vi "light sensor.vi"() -> ()   [LabVIEW 2019]
uses:
  <vilib>/MakerHub/LINX/Public/Utilities/Open Serial.vi
  <vilib>/MakerHub/LINX/LMH-LINX.lvlib
panel:
  out "dt":u32
  out "Lux value":dbl(graph)
  out "current 16bit sensor value":u16
  out "I2C Channel (0)":u8=4
  out "Device Name":string
  in  "stop":bool
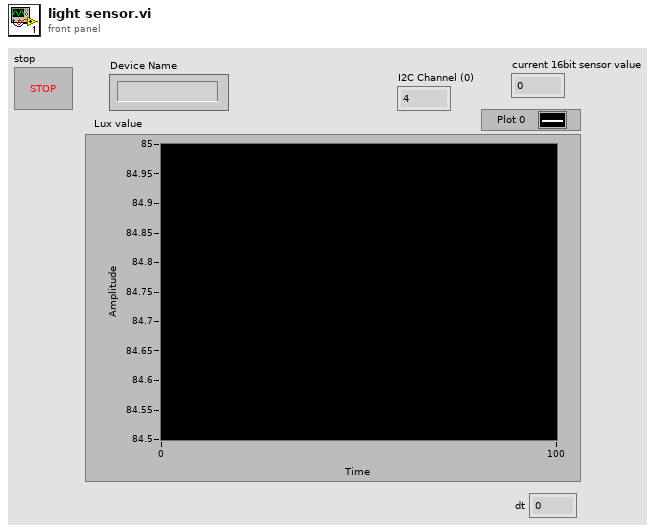
[diagram p1: front panel]
types:
  T1 = typedef "LMH-LINX.lvlib/LINX Ref.ctl" = cluster{"IO":T2, "Interface":T3, "LINX Device Config":T4}
  T2 = typedef "LMH-LINX.lvlib/Platform.ctl" = enum16{"Remote", "Local"}
  T3 = typedef "LMH-LINX.lvlib/Interface.ctl" = enum16{"Serial", "TCP"}
  T4 = typedef "LMH-LINX.lvlib/Device.lvlib/LINX Device Config.ctl" = cluster{"Interface":T3, "COM Port":refnum<visa-resource-name>, "TCP Configuration":T5, "Device Family":u8, "Device ID":u8, "Device Name":string, "TCP Ref":refnum<k5>, "Channels":T6}
  T5 = typedef "LMH-LINX.lvlib/Device.lvlib/TCP Config.ctl" = cluster{"IP Address":string, "Port":u16}
  T6 = typedef "LMH-LINX.lvlib/Channels.ctl" = cluster{"DI":u8[], "DO":u8[], "AI":u8[], "AO":u8[], "PWM":u8[], "QE":u8[], "UART":u8[], "I2C 2":u8[], "SPI":u8[], "CAN":u8[], "Servo":u8[], "AI Ref (V)":dbl, "AI Resolution (Bits)":u8, "AO Ref (V)":dbl, "AO Resolution (Bits)":u8}
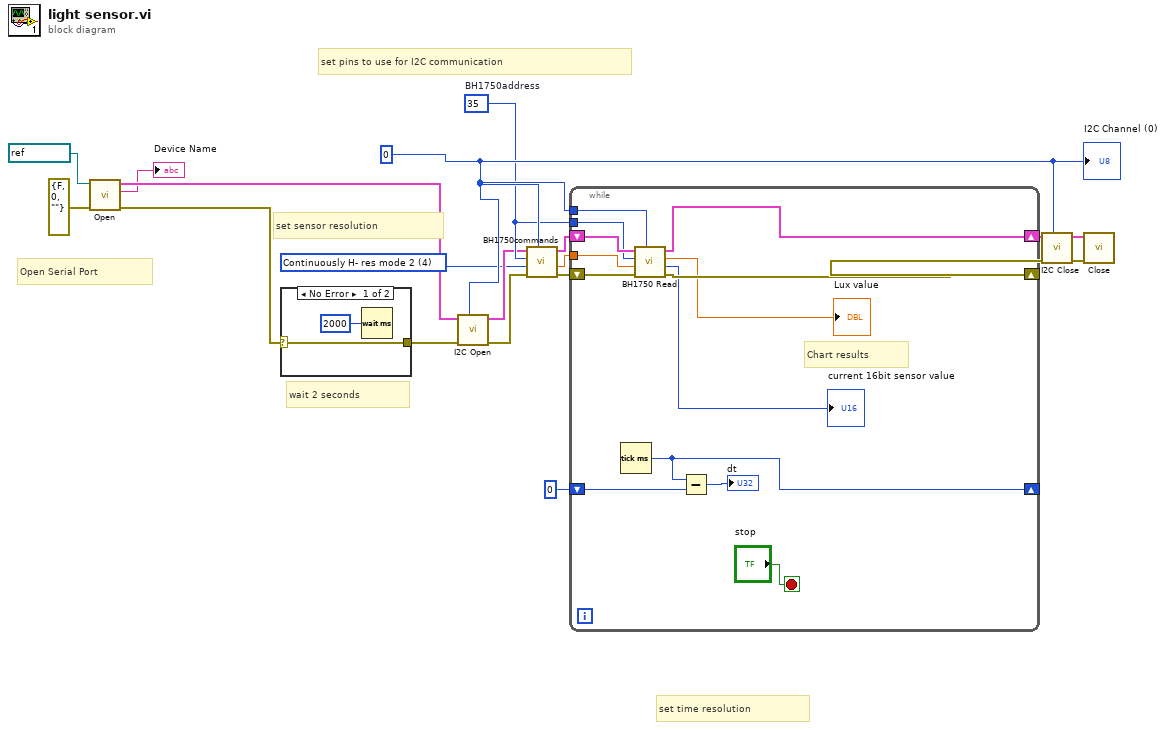
[diagram p0: block diagram]
diagram:
  w3 = u16 4 items=["power down", "Power on", "Reset", "Continuously H- res", "Continuously H- res mode 2", "Continuously L- res", "One time H- res ", "One time H- res mode 2", "One time L res ", "Change Measurement time High bit", "Change Measurement time  Low Bit"] ("Command")
  w7 = u8 35  # BH1750address
  w8 = u8 0 ("I2C Channel (0)")
  # "set pins to use for I2C communication"
  # "set sensor resolution"
  # "wait 2 seconds"
  # "Open Serial Port"
  # "set time resolution"
  n1 = call-poly <vilib>:"Open.vi"("Error In"=errorcluster {"status"=FALSE, "code"=0, "source"=""}, "Serial Port"=refnum<visa-resource-name> "COM3") -> ("Error Out"=w13:errorcluster, "Device Name"=→"Device Name":string, "LINX Resource"=w17:T1)  [unwired: 7 in]
  n2 = case shown="No Error" w13 {
    selector: w13 -> [w20 w22]
    tunnel: [w20 w22] -> w12
    frame No Error {
      n3 = Wait (ms)(milliseconds to wait=u32 2000) -> ()  [unwired: 1 out]
    }
    frame Error {
    }
  }
  n4 = call <vilib>:"I2C Open.vi"("I2C Channel (0)"=w8, "Error In"=w12, "LINX Resource"=w17) -> ("Error Out"=w5:errorcluster, "LINX Resource"=w6:T1)  [unwired: 7 in]
  n5 = call "BH1750commands.vi"("I2C Channel"=w8, "Error In"=w5, "Command"=w3, "I2C Slave Address (0)"=w7, "LINX Resource"=w6) -> ("Error Out"=w4:errorcluster, "Resoultion (lux)"=w1:dbl, "LINX Resource out"=w9:T1)  [unwired: 4 in]
  n6 = while {
    tunnel: w8 -> [w23]
    shift-right: [w35] -> w19
    shift-left: w9 -> [w26]
    shift-right: [w33] -> w18
    shift-left: w4 -> [w34]
    tunnel: w7 -> [w24]
    shift-right: [w31] -> _
    shift-left: u32 0 ("millisecond timer value") -> [w30]
    tunnel: w1 -> [w25]
    stop <- "stop" stop-if-true
    # "Chart results"
    n7 = Tick Count (ms)() -> (millisecond timer value=w31:u32)
    n8 = call "BH1750 Read.vi"("I2C Channel (0)"=w23, "error in (no error)"=w34, "Resoultion (lux)"=w25, "BH1750address"=w24, "LINX Resource in"=w26) -> ("error out"=w33:errorcluster, "64 bit value"=→"current 16bit sensor value":u16, "Lux value"=→"Lux value":dbl, "LINX Resource"=w35:T1)  [unwired: 3 in]
    n9 = Subtract(x=w31, y=w30) -> (x-y=→"dt":u32)
  }
  n10 = call <vilib>:"I2C Close.vi"("I2C Channel (0)"=w8, "Error In"=w18, "LINX Resource"=w19) -> ("Error Out"=w11:errorcluster, "LINX Resource"=w15:T1)  [unwired: 7 in]
  n11 = call <vilib>:"Close.vi"("Error In"=w11, "LINX Resource"=w15) -> ()  [unwired: 9 in, 1 out]
  "I2C Channel (0)" <- w8
